vi "lectura corriente.vi"(4 "read buffer":string) -> (0 "Corriente motor3":dbl[](array[numeric]), 1 "Corriente motor2":dbl[](array[numeric]), 2 "Corriente motor1":dbl[](array[numeric]))   [LabVIEW 2020]
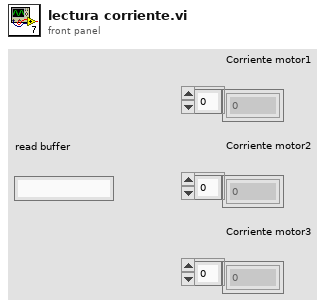
[diagram p1: front panel]
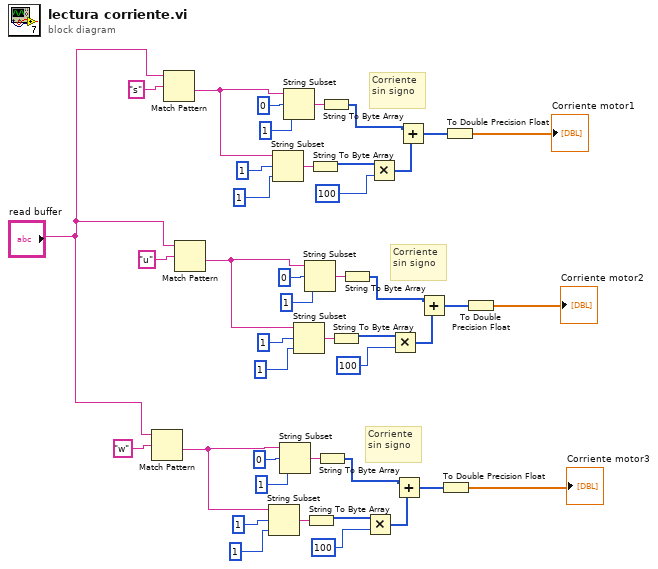
[diagram p0: block diagram]
diagram:
  # "Corriente sin signo"
  # "Corriente sin signo"
  # "Corriente sin signo"
  n1 = Match Pattern(string="read buffer", regular expression="w") -> (after substring=w37:string)  [unwired: 1 in, 3 out]
  n2 = Match Pattern(string="read buffer", regular expression="s") -> (after substring=w13:string)  [unwired: 1 in, 3 out]
  n3 = Match Pattern(string="read buffer", regular expression="u") -> (after substring=w25:string)  [unwired: 1 in, 3 out]
  n4 = String Subset(string=w37, offset (0)=1, length (rest)=1 ("length (rest)")) -> (substring=w30:string)
  n5 = String Subset(string=w13, offset (0)=1, length (rest)=1 ("length (rest)")) -> (substring=w4:string)
  n6 = String Subset(string=w37, offset (0)=0, length (rest)=1 ("length (rest)")) -> (substring=w29:string)
  n7 = String Subset(string=w13, offset (0)=0, length (rest)=1 ("length (rest)")) -> (substring=w3:string)
  n8 = String Subset(string=w25, offset (0)=1, length (rest)=1 ("length (rest)")) -> (substring=w18:string)
  n9 = String Subset(string=w25, offset (0)=0, length (rest)=1 ("length (rest)")) -> (substring=w17:string)
  n10 = String To Byte Array(string=w30) -> (unsigned byte array=w32:u8[])
  n11 = String To Byte Array(string=w4) -> (unsigned byte array=w7:u8[])
  n12 = String To Byte Array(string=w29) -> (unsigned byte array=w34:u8[])
  n13 = String To Byte Array(string=w3) -> (unsigned byte array=w10:u8[])
  n14 = String To Byte Array(string=w18) -> (unsigned byte array=w20:u8[])
  n15 = String To Byte Array(string=w17) -> (unsigned byte array=w22:u8[])
  n16 = Multiply(x=w32, y=100) -> (x*y=w33:i32[])
  n17 = Multiply(x=w7, y=100) -> (x*y=w9:i32[])
  n18 = Multiply(x=w20, y=100) -> (x*y=w21:i32[])
  n19 = Add(x=w34, y=w33) -> (x+y=w35:i32[])
  n20 = Add(x=w10, y=w9) -> (x+y=w11:i32[])
  n21 = Add(x=w22, y=w21) -> (x+y=w23:i32[])
  n22 = To Double Precision Float(number=w35) -> (double precision float=→"Corriente motor3":dbl[])
  n23 = To Double Precision Float(number=w11) -> (double precision float=→"Corriente motor1":dbl[])
  n24 = To Double Precision Float(number=w23) -> (double precision float=→"Corriente motor2":dbl[])
